vi "FTW-JSON-ObjectManip-AddPair.vi"(0 "Input JSON Object":string, 5 "Key":string, 7 "Value":string, 11 "error in":errorcluster) -> (4 "Output JSON Object":string, 15 "error out":errorcluster)   [LabVIEW 2014]
panel:
  # "Inputs"
  # "Outputs"
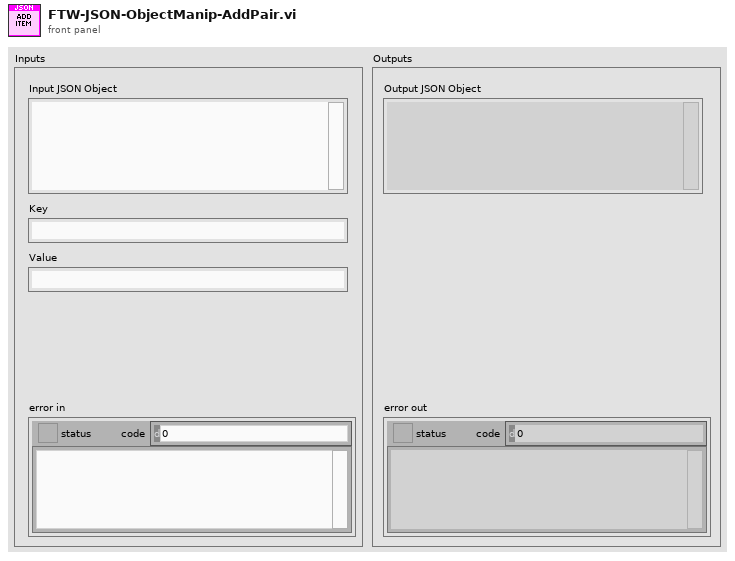
[diagram p1: front panel]
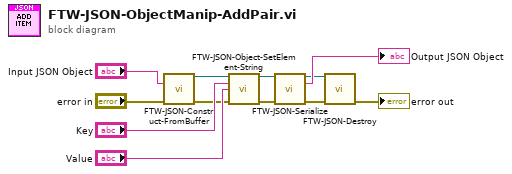
[diagram p0: block diagram]
diagram:
  n1 = call "FTW-JSON-Construct-FromBuffer.vi"("JSON String (UTF-8)"="Input JSON Object", "error in"="error in") -> ("JSON Object"=w4:refnum<data-value>, "error out"=w2:errorcluster)  [unwired: 12 in]
  n2 = call "FTW-JSON-Object-SetElement-String.vi"("JSON Object"=w4, "Key"="Key", "Value"="Value", "error in"=w2) -> ("JSON Object out"=w3:refnum<class "FTW-JSON.lvclass">, "error out"=w1:errorcluster)  [unwired: 10 in]
  n3 = call "FTW-JSON-Serialize.vi"("JSON Object"=w3, "error in"=w1) -> ("JSON Object out"=w6:refnum<class "FTW-JSON.lvclass">, "JSON String (UTF-8)"=→"Output JSON Object":string, "error out"=w5:errorcluster)  [unwired: 11 in]
  n4 = call "FTW-JSON-Destroy.vi"("JSON Object"=w6, "error in"=w5) -> ("error out"=→"error out":errorcluster)  [unwired: 13 in]
